vi "Read Configuration.vi"(7 "Type and Defaults":variant, 8 "error in (no error)":errorcluster, 11 "JSON Config File in":refnum<class "JSON Config File.lvclass">) -> (0 "error out":errorcluster, 2 "Configuration":variant, 3 "JSON Config File out":refnum<class "JSON Config File.lvclass">)   [LabVIEW 2019, in "JSON Config File.lvclass"]
doc: "JKI JSON 1.1.10.37\nTomi Maila - JKI\nCopyright (c) 2017, JKI"
uses:
  JSON Config File.lvclass
  JSON Config File.lvclass/JSON Config File.ctl
  vi.lib/addons/_JKI.lib/Serialization/JSON/JKI JSON Serialization.lvlib
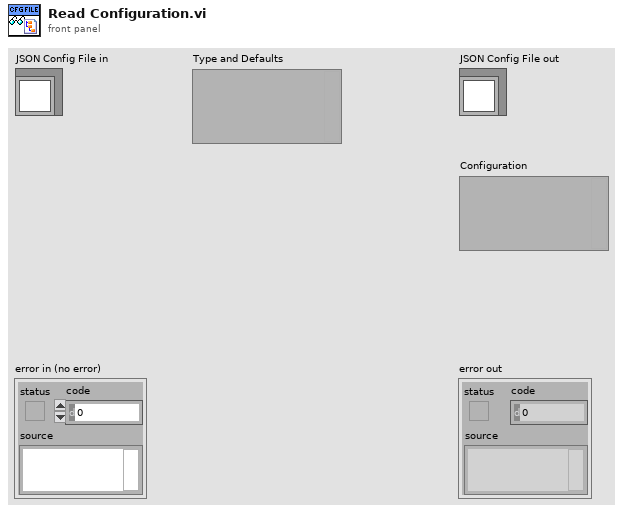
[diagram p1: front panel]
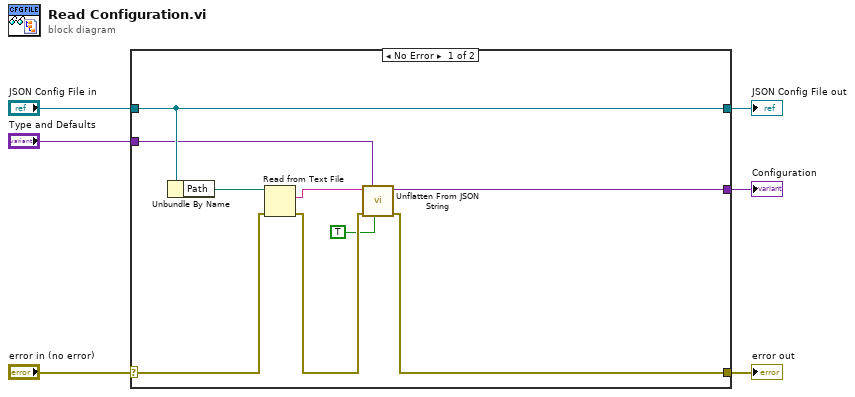
[diagram p0: block diagram]
diagram:
  n1 = case shown="No Error" "error in (no error)" {
    selector: "error in (no error)" -> [w13 w17]
    tunnel: [w9 w17] -> w5
    tunnel: [w15 w16] -> w3
    tunnel: "JSON Config File in" -> [w15 w16]
    tunnel: "Type and Defaults" -> [w11 _]
    tunnel: [w7 _] -> w1
    frame No Error {
      n2 = Unbundle By Name(w15) -> ("Path"=w14:path)
      n3 = Read from Text File(file (use dialog)=w14, error in=w13) -> (text=w12:string, error out=w10:errorcluster)  [unwired: 2 in, 2 out]
      n4 = call "Unflatten From JSON String.vi"("Nulls as Defaults (F)"=TRUE, "Type and Defaults"=w11, "error in (no error)"=w10, "JSON String"=w12) -> ("error out"=w9:errorcluster, "Variant"=w7:variant)  [unwired: 6 in]
    }
    frame Error {
    }
  }
  "error out" <- w5
  "JSON Config File out" <- w3
  "Configuration" <- w1
